vi "Waveform.vi"() -> ()   [LabVIEW 2020]
panel:
  in  "Array":waveform(dbl)[](array[waveform])
  out "Waveform Graph":waveform(dbl)[](graph)
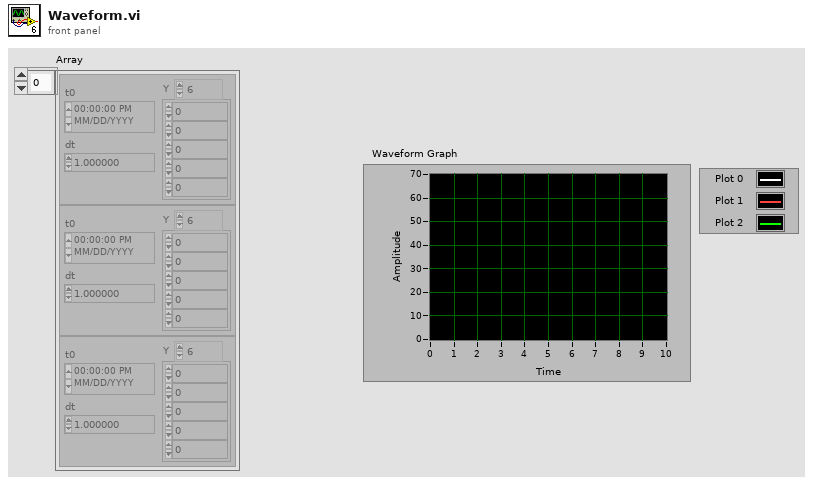
[diagram p1: front panel]
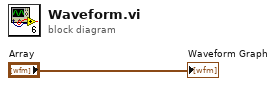
[diagram p0: block diagram]
diagram:
  "Waveform Graph" <- "Array"
